vi "Write Controls.vi"(5 "Controls":refnum<class "Control.lvclass">[](array[class]), 9 "Pane in":refnum<class "Pane.lvclass">) -> (3 "Pane out":refnum<class "Pane.lvclass">)   [LabVIEW 2014, in "Pane.lvclass"]
uses:
  Pane.lvclass
  Control/Control.lvclass
  Pane.lvclass/Pane.ctl
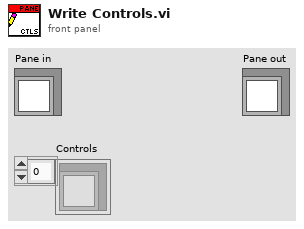
[diagram p1: front panel]
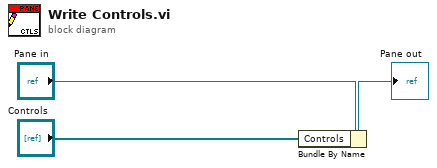
[diagram p0: block diagram]
diagram:
  n1 = Bundle By Name(cluster="Pane in", "Controls"="Controls") -> (→"Pane out":refnum<class "Pane.lvclass">)
